vi "ScreeningPlatform_v4.vi"() -> ()   [LabVIEW 2018]
uses:
  <instrlib>/Chemyx/_driver/Basic driver/Communication/controls/comm_rate_enum.ctl
  <vilib>/Utility/file.llb/Read Delimited Spreadsheet (DBL).vi
  <vilib>/Utility/file.llb/Read Delimited Spreadsheet (string).vi
  <vilib>/regexp/Match Regular Expression.xnode
  <instrlib>/Chemyx/_driver/Chemyx_Syringe_Pump_driver.lvlib
panel:
  out "Start Scan":dbl format="%#_1f"
  out "Stop Scan":dbl format="%#_1f"
  in  "stop":bool
  in  "GPC Injections":bool=TRUE
  out "Comments file":path=path "Z:/Sci-Chem/PRD/NMR 112/Automated Platform/2020/08/17/332PM_JOreneosdjf/Software Details/JOreneosdjf_Comments.txt"
  in  "Insert Comment":bool
  in  "Cooment":string
  out "NMR use":bool
  out "GPC use":bool
  out "GPC Dead Volume":bool
  out "GPC timesweep":bool
  out "NMR timesweep":bool
  out "NMR Dead Volume":bool
  out "Stabilisation":bool
  out "OverviewTextFile":path=path "Z:/Sci-Chem/PRD/NMR 112/Automated Platform/2020/08/17/332PM_JOreneosdjf/Software Details/JOreneosdjf_OverviewText.txt"
  out "To... (min)":dbl
  out "From.. (min)":dbl
  out "Dead Volume 3":dbl
  out "Dilution Flowrate":dbl
  out "NMR interval":dbl
  out "Dead Volume 1":dbl
  out "Stabilisation Factor":dbl
  out "Reactor Volume":dbl
  out "Dead Volume 2":dbl
  out "GPC interval":dbl
  out "TimesweepStringArray":string[][](array[string])=[["1.0", "5.0", "1.0", "1.0", "0.2", "1.3", "0.43", "0.26", "3", "0.157", "1.5", "2.15", "1.3", "0.10466666666666667", "15", "GPCandNMR"]]
  out "Experiment started":bool
  out "Experiment folder created":bool
  out "Experiment found":bool
  in  "Tab Control":enum32{"Overview", "Details", "Folders"}(tab)=enum."Folders"
  in  "Listbox":i32(listbox)
  in  "Finished_timesweeps":i32(listbox)=-1
  out "Timesweep queue":string[](array[string])=["Timesweep 1: From 1.0 minutes (1.000 mL/min) to 5.0 minutes (0.200 mL/min) with GPC intervals of 3.0 minutes."]
  out "Content Textfile":string
  out "Experiment Folder (path)":path=path "Z:/Sci-Chem/PRD/NMR 112/Automated Platform/2020/09/30/936AM_2"
  out "Mode":string
  out "TimesweepArray":dbl[][](array[numeric])
  out "Last Comment":string
  in  "Python Communication Folder":path=path "S:/Sci-Chem/PRD/NMR 112/Automated Platform/Final_LabView_allVIs/PythonCommunication"
  in  "Where to save?":path=path "S:/Sci-Chem/PRD/NMR 112/Automated Platform"
  out "Status injections":string="Waiting for injection 0"
  out "NAME":string="No new experiment found..."
  out "output array":dbl[](array[numeric])=[5.0, 17.0]
  out "Reaction":dbl[][](array[numeric])
  out "Next injection":u8(slide) scale=0.0..100.0
  out "GPC Samples":dbl format="%#_1f"
  in  "GPC connection port 2":refnum<visa-resource-name>
  in  "Pump":refnum<visa-resource-name>="COM11"
  out "Waiting NMR":dbl format="%#_2g"
  out "Waiting GPC":dbl format="%#_2f"
  out "scan":i32
  out "GPC Status":string
  out "NMR Status":string
  out "Current timesweep":i32
  out "Stabilisation time (min)":dbl=nan format="%#_2g"
  out "Stabilisation time (sec)":dbl=nan
  out "GPC Timesweep":u8(slide) scale=0.0..100.0
  out "NMR Timesweep bar":u8(slide) scale=0.0..100.0
  out "StabilisationBar":u8(slide) scale=0.0..100.0
  out "Status":string="Start program..."
  # "Reactor Volume"
  # "mL"
  # "Dead Volume 2"
  # "mL"
  # "Dead Volume 1"
  # "mL"
  # "Dead Volume 3"
  # "mL"
  # "Stabilisation Factor"
  # "x"
  # "Dilution Flowrate"
  # "mL/min"
  # "NMR interval"
  # "sec"
  # "GPC interval"
  # "min"
  # "Stabilisation"
  # "min"
  # "Use"
  # "Dead Volume"
  # "Timesweep"
  # "Done"
  # "Status"
  # "Number"
  # "min"
  # "NMR"
  # "min"
  # "GPC"
  # "Next injection"
  # "Comment"
  # "scan"
  # "to"
  # "Experiment found"
  # "Experiment folder created"
  # "Experiment started"
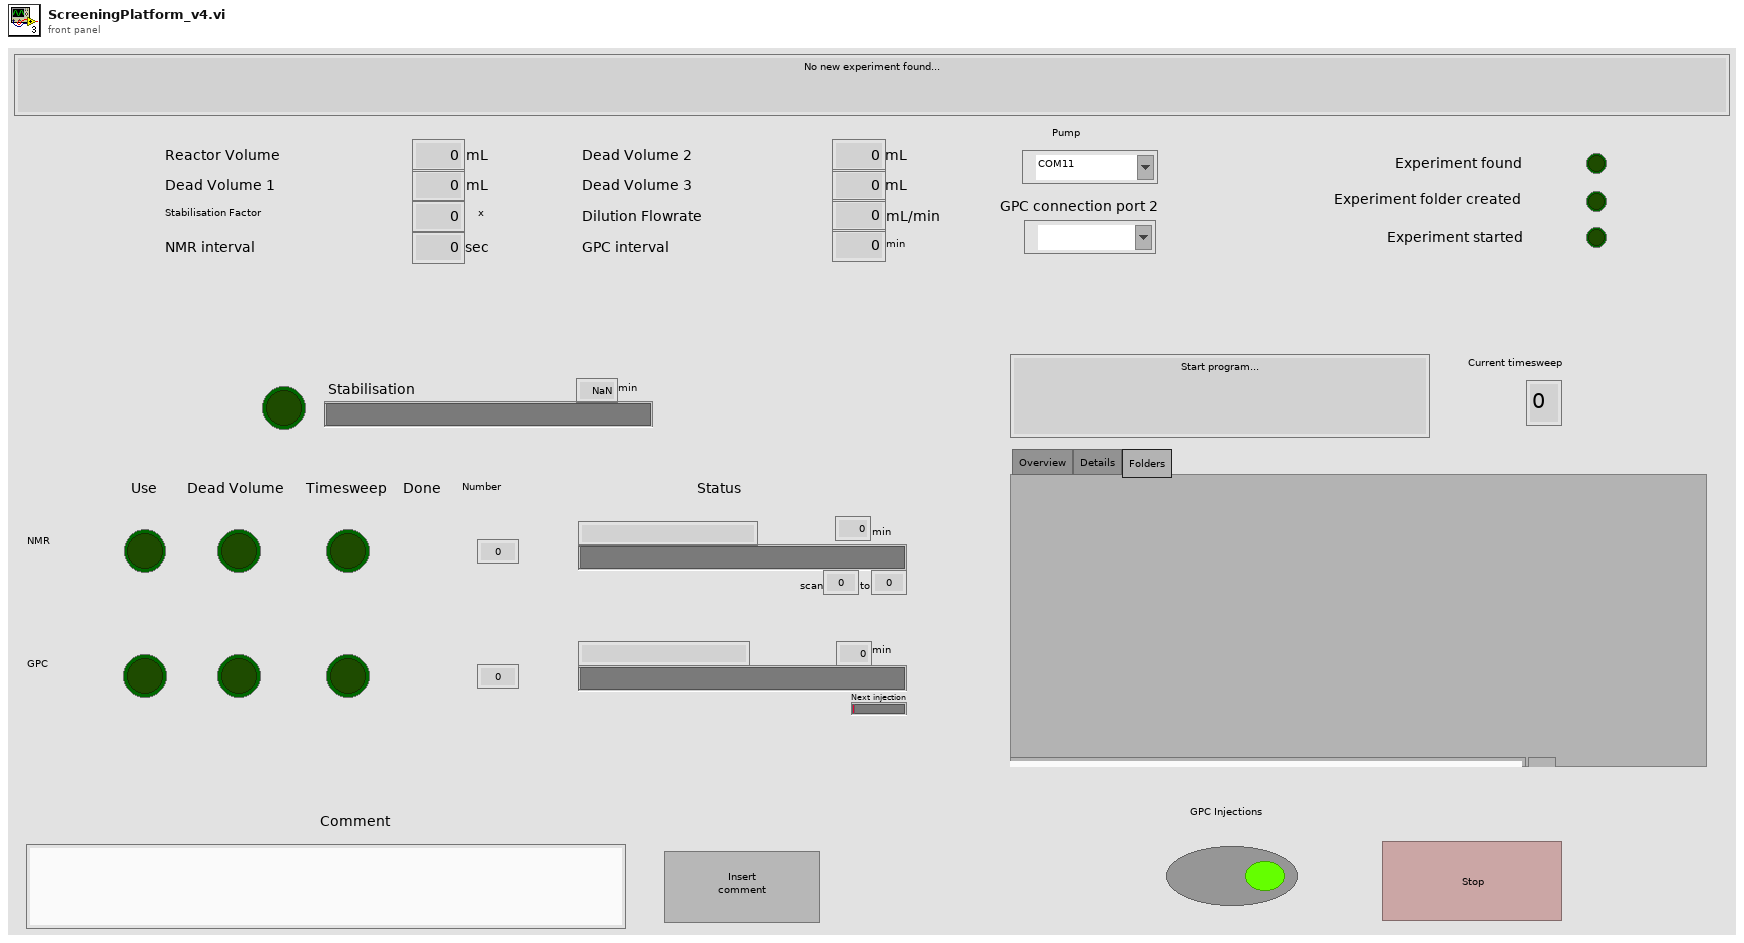
[diagram p1: front panel]
types:
  T1 = typedef "Chemyx_Syringe_Pump_driver.lvlib/comm_rate_enum.ctl" = enum16{"9600", "38400"}
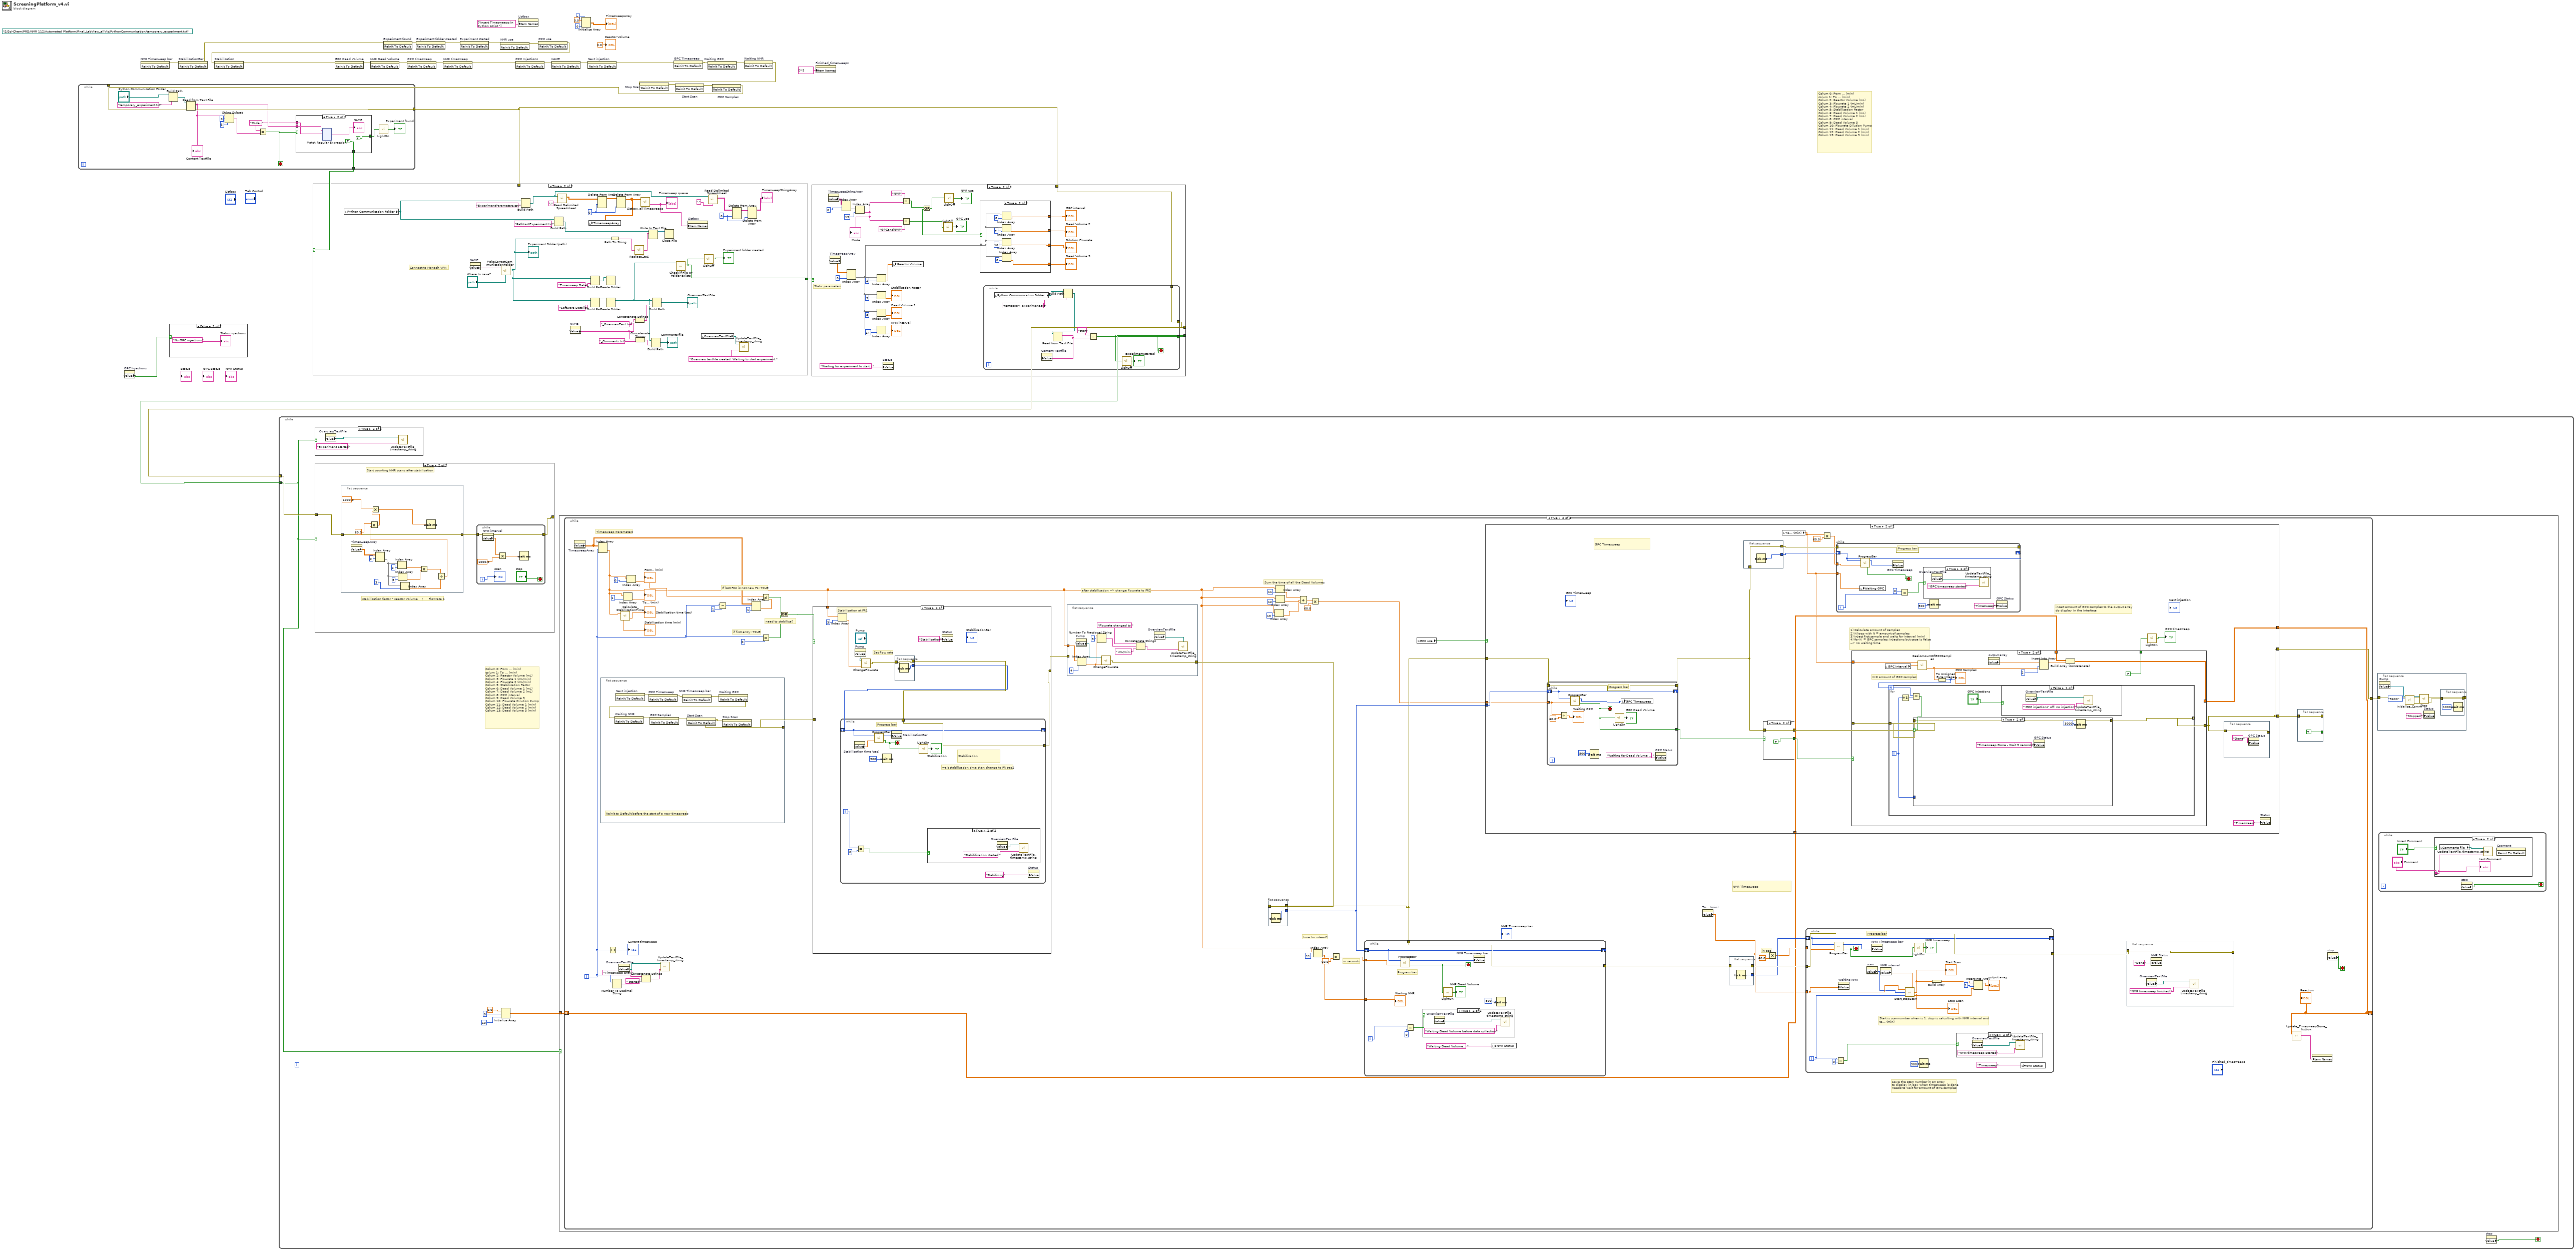
[diagram p0: block diagram]
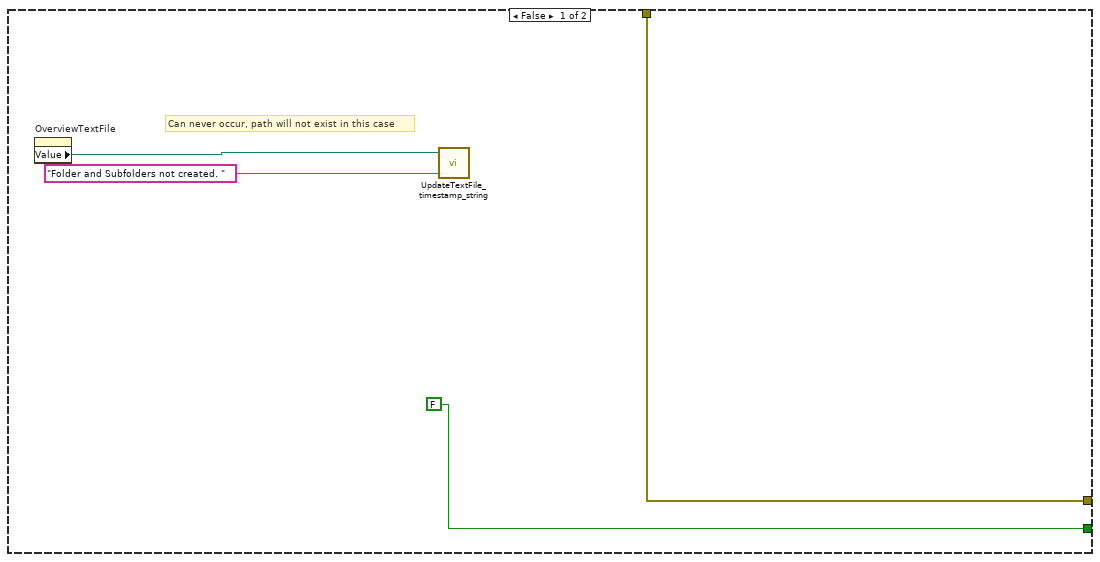
[diagram p3: hidden frame]
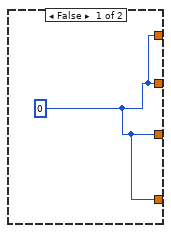
[diagram p4: hidden frame]
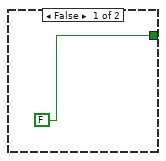
[diagram p5: hidden frame]
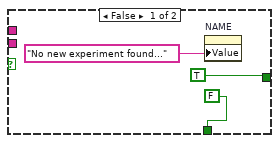
[diagram p6: hidden frame]
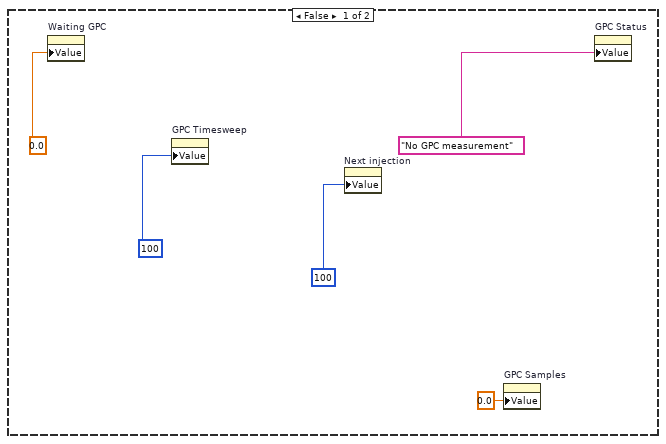
[diagram p11: hidden frame]
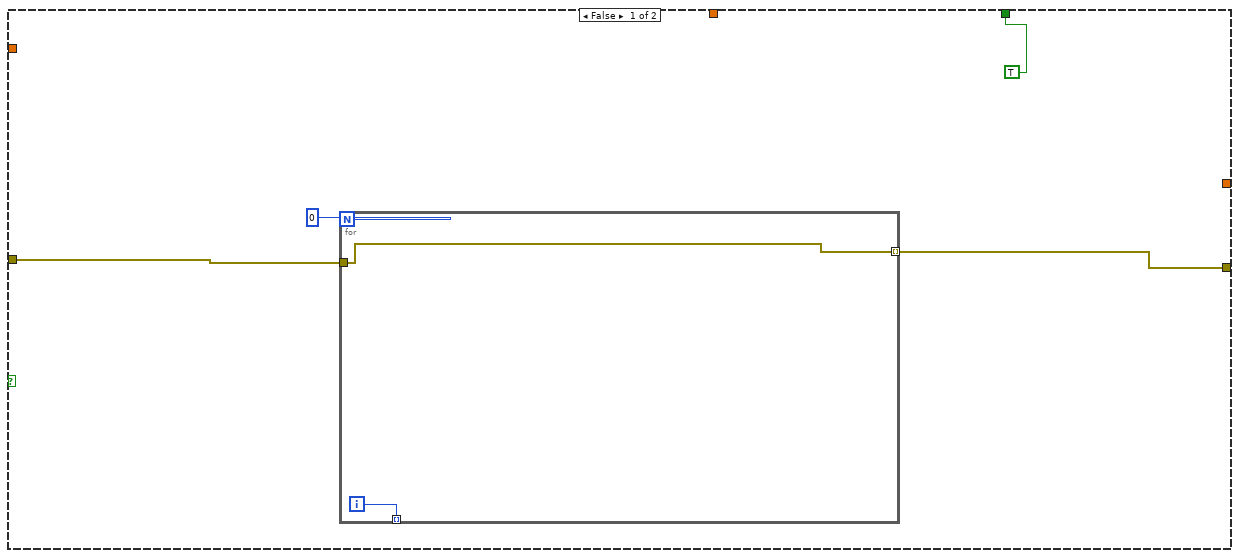
[diagram p12: hidden frame]
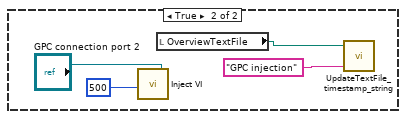
[diagram p13: hidden frame]
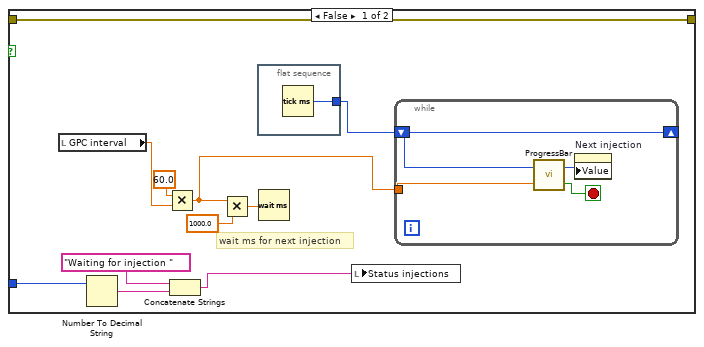
[diagram p14: hidden frame]
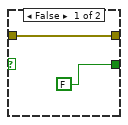
[diagram p16: hidden frame]
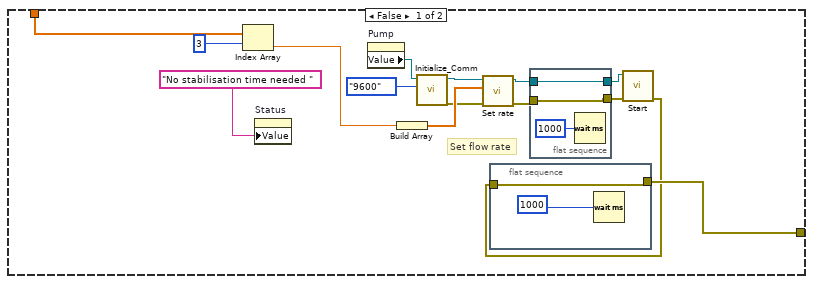
[diagram p18: hidden frame]
diagram:
  (unwired) path "S:/Sci-Chem/PRD/NMR 112/Automated Platform/Final_LabView_allVIs/PythonCommunication/temporary_experiment.txt" ("file path (dialog if empty)")
  # "Colum 0: From ... (min)\ncolum 1: To ... (min)\nColum 2: Reactor Volume (mL)\nColum 3: Flowrate 1 (mL/min)\nColum 4: Flowrate 2 (mL/min)\nColum 5: Stabilisation Factor\nColum 6: Dead Volume 1 (mL)\nColum 7: Dead Volume 2 (mL)\nColum 8: GPC interval\nColum 9: Dead Volume 3\nColum 10: Flowrate Dilution Pump\nColum 11: Dead Volume 1 (min)\nColum 12: Dead Volume 2 (min)\nColum 13: Dead Volume 3 (min)"
  n1 = property on="GPC Injections" class="Bool (strict)"() -> ("Value"=w28:bool)  [unwired: 2 in, 2 out]
  n2 = invoke on="NMR Timesweep bar" class="Slide (strict)" method="Reinit To Default"() -> (error out=w30:errorcluster)  [unwired: 3 in, 2 out]
  n3 = case shown="False" w28 {
    frame False {
      "Status injections" <- "No GPC injections"
    }
    frame True {
    }
  }
  n4 = invoke on="StabilisationBar" class="Slide (strict)" method="Reinit To Default"(error in=w30) -> (error out=w25:errorcluster)  [unwired: 2 in, 2 out]
  n5 = invoke on="Experiment found" class="Bool (strict)" method="Reinit To Default"(error in=w25) -> (error out=w27:errorcluster)  [unwired: 2 in, 2 out]
  n6 = invoke on="Experiment folder created" class="Bool (strict)" method="Reinit To Default"(error in=w27) -> (error out=w26:errorcluster)  [unwired: 2 in, 2 out]
  n7 = invoke on="Experiment started" class="Bool (strict)" method="Reinit To Default"(error in=w26) -> (error out=w3:errorcluster)  [unwired: 2 in, 2 out]
  n8 = invoke on="NMR use" class="Bool (strict)" method="Reinit To Default"(error in=w3) -> (error out=w2:errorcluster)  [unwired: 2 in, 2 out]
  n9 = property on="Listbox" class="LstBox (strict)"("Item Names"=string[] ["Insert Timesweeps in Python script "]) -> ()  [unwired: 2 in, 2 out]
  n10 = invoke on="GPC use" class="Bool (strict)" method="Reinit To Default"(error in=w2) -> (error out=w1:errorcluster)  [unwired: 2 in, 2 out]
  n11 = invoke on="Stabilisation" class="Bool (strict)" method="Reinit To Default"(error in=w1) -> (error out=w24:errorcluster)  [unwired: 2 in, 2 out]
  n12 = invoke on="GPC Dead Volume" class="Bool (strict)" method="Reinit To Default"(error in=w24) -> (error out=w23:errorcluster)  [unwired: 2 in, 2 out]
  n13 = invoke on="NMR Dead Volume" class="Bool (strict)" method="Reinit To Default"(error in=w23) -> (error out=w22:errorcluster)  [unwired: 2 in, 2 out]
  n14 = invoke on="GPC timesweep" class="Bool (strict)" method="Reinit To Default"(error in=w22) -> (error out=w21:errorcluster)  [unwired: 2 in, 2 out]
  n15 = invoke on="NMR timesweep" class="Bool (strict)" method="Reinit To Default"(error in=w21) -> (error out=w18:errorcluster)  [unwired: 2 in, 2 out]
  n16 = invoke on="GPC Injections" class="Bool (strict)" method="Reinit To Default"(error in=w18) -> (error out=w20:errorcluster)  [unwired: 2 in, 2 out]
  n17 = invoke on="NAME" class="Str" method="Reinit To Default"(error in=w20) -> (error out=w19:errorcluster)  [unwired: 2 in, 2 out]
  n18 = Initialize Array(0.0 ("element"), 0 ("dimension size"), 0 ("dimension size")) -> (→"TimesweepArray":dbl[][])
  n19 = invoke on="Next injection" class="Slide (strict)" method="Reinit To Default"(error in=w19) -> (error out=w13:errorcluster)  [unwired: 2 in, 2 out]
  n20 = invoke on="GPC Timesweep" class="Slide (strict)" method="Reinit To Default"(error in=w13) -> (error out=w15:errorcluster)  [unwired: 2 in, 2 out]
  n21 = invoke on="Waiting GPC" class="DigNum (strict)" method="Reinit To Default"(error in=w15) -> (error out=w16:errorcluster)  [unwired: 2 in, 2 out]
  n22 = invoke on="Waiting NMR" class="DigNum (strict)" method="Reinit To Default"(error in=w16) -> (error out=w12:errorcluster)  [unwired: 2 in, 2 out]
  n23 = invoke on="Stop Scan" class="DigNum (strict)" method="Reinit To Default"(error in=w12) -> (error out=w17:errorcluster)  [unwired: 2 in, 2 out]
  n24 = invoke on="Start Scan" class="DigNum (strict)" method="Reinit To Default"(error in=w17) -> (error out=w14:errorcluster)  [unwired: 2 in, 2 out]
  n25 = invoke on="GPC Samples" class="DigNum (strict)" method="Reinit To Default"(error in=w14) -> (error out=w11:errorcluster)  [unwired: 2 in, 2 out]
  n26 = while {
    tunnel: [w49] -> w34
    tunnel: w11 -> [w42]
    tunnel: [w41] -> w29
    stop <- w45 stop-if-true
    w43 = "Code,," ("y")
    n27 = Build Path(base path="Python Communication Folder", name or relative path="temporary_experiment.txt") -> (appended path=w36:path)
    n28 = Read from Text File(file (use dialog)=w36, error in=w42) -> (text=w44:string, error out=w49:errorcluster)  [unwired: 2 in, 2 out]
    "Content Textfile" <- w44
    n29 = String Subset(string=w44, offset (0)=0, length (rest)=6 ("length (rest)")) -> (substring=w46:string)
    n30 = Equal?(x=w43, y=w46) -> (x = y?=w45:bool)
    n31 = case shown="True" w45 {
      tunnel: w44 -> [_ w57]
      tunnel: w43 -> [_ w56]
      tunnel: [FALSE TRUE] -> w41
      tunnel: [TRUE FALSE] -> w40
      frame False {
        n32 = property on="NAME" class="Str"("Value"="No new experiment found...") -> ()  [unwired: 2 in, 2 out]
      }
      frame True {
        n33 = xnode "Match Regular Expression"("input string"=w57, "regular expression"=w56) -> ("after match"=→"NAME":string)  [unwired: 4 in, 4 out]
      }
    }
    n34 = call "LightOn.vi"("Turns off when..."=w40) -> ("Light Indicator"=→"Experiment found":bool)
  }
  n35 = case shown="True" w29 {
    tunnel: w34 -> [_ _]
    tunnel: [FALSE w198] -> w31
    frame False {
    }
    frame True {
      w191 = 0 ("index (row)")
      w208 = 0 ("length")
      # "Connect to Monash VPN"
      n36 = local read "Python Communication Folder"() -> (w177:path)
      n37 = property on="NAME" class="Str"() -> ("Value"=w203:string)  [unwired: 2 in, 2 out]
      n38 = call "MakeCorrectCommunicationFolder.vi"("Main_dataFolder"="Where to save?", "SampleName"=w203) -> ("Communication Folder"=w182:path)  [unwired: 1 out]
      "Experiment Folder (path)" <- w182
      n39 = Build Path(base path=w177, name or relative path="ExperimentParameters.csv") -> (appended path=w179:path)
      n40 = Build Path(base path=w177, name or relative path="PathLastExperiment.txt") -> (appended path=w180:path)
      n41 = call-poly <vilib>:"Read Delimited Spreadsheet.vi"("file path (dialog if empty)"=w179, "delimiter (\\t)"="," ("delimiter (\\t)")) -> ("all rows"=w207:dbl[][])  [unwired: 8 in, 5 out]
      n42 = property on="NAME" class="Str"() -> ("Value"=w188:string)  [unwired: 2 in, 2 out]
      n43 = Build Path(base path=w182, name or relative path="Timesweep Data") -> (appended path=w199:path)
      n44 = Build Path(base path=w182, name or relative path="Software Details") -> (appended path=w200:path)
      n45 = Delete From Array(array=w207, index (row)=w208) -> (array with subset deleted=w209:dbl[][])  [unwired: 2 in, 1 out]
      n46 = Create Folder(path (use dialog)=w199) -> ()  [unwired: 2 in, 3 out]
      n47 = Create Folder(path (use dialog)=w200) -> (created path=w189:path)  [unwired: 2 in, 2 out]
      n48 = Path To String(path=w182) -> (string=w175:string)
      n49 = Delete From Array(array=w209, index (col)=w208) -> (array with subset deleted=w183:dbl[][])  [unwired: 2 in, 1 out]
      n50 = local write "TimesweepArray"(w183) -> ()
      n51 = call "ReplaceZtoS.vi"("String"=w175) -> ("result string"=w174:string)
      n52 = Concatenate Strings(w188, "_OverviewText.txt" ("string")) -> (w201:string)
      n53 = Concatenate Strings(w188, "_Comments.txt" ("string")) -> (w186:string)
      n54 = call "Listbox_allTimesweeps.vi"("new array"=w183) -> ("output array"=w184:string[])  [unwired: 1 out]
      "Timesweep queue" <- w184
      n55 = Write to Text File(file (use dialog)=w180, text=w174) -> (refnum out=w205:refnum<file>)  [unwired: 2 in, 2 out]
      n56 = Build Path(base path=w189, name or relative path=w186) -> (appended path=→"Comments file":path)
      n57 = Build Path(base path=w189, name or relative path=w201) -> (appended path=→"OverviewTextFile":path)
      n58 = Close File(refnum=w205) -> ()  [unwired: 1 in, 2 out]
      n59 = call <vilib>:"Check if File or Folder Exists.vi"("path"=w189) -> ("file or folder exists?"=w198:bool)  [unwired: 8 in, 2 out]
      n60 = property on="Listbox" class="LstBox (strict)"("Item Names"=w184) -> ()  [unwired: 2 in, 2 out]
      n61 = local read "OverviewTextFile"() -> (w173:path)
      n62 = call "LighOff.vi"("Turns on when..."=w198) -> ("Light Indicator"=→"Experiment folder created":bool)
      n63 = call-poly <vilib>:"Read Delimited Spreadsheet.vi"("file path (dialog if empty)"=w179, "delimiter (\\t)"="," ("delimiter (\\t)")) -> ("all rows"=w194:string[][])  [unwired: 8 in, 5 out]
      n64 = Delete From Array(array=w194, index (row)=w191) -> (array with subset deleted=w193:string[][])  [unwired: 2 in, 1 out]
      n65 = call "UpdateTextFile_timestamp_string.vi"("string"="Overview textfile created. Waiting to start experiment.", "file path"=w173) -> ()  [unwired: 1 in]
      n66 = Delete From Array(array=w193, index (col)=w191) -> (array with subset deleted=→"TimesweepStringArray":string[][])  [unwired: 2 in, 1 out]
    }
  }
  n67 = case shown="True" w31 {
    tunnel: [w214 w245] -> w33
    tunnel: [FALSE w244] -> w32
    tunnel: w34 -> [w214 w243]
    frame False {
      # "Can never occur, path will not exist in this case"
      n68 = property on="OverviewTextFile" class="Path"() -> ("Value"=w212:path)  [unwired: 2 in, 2 out]
      n69 = call "UpdateTextFile_timestamp_string.vi"("string"="Folder and Subfolders not created. ", "file path"=w212) -> ()  [unwired: 1 in]
    }
    frame True {
      # "Static parameters"
      n70 = property on="TimesweepStringArray" class="Arr (strict)"() -> ("Value"=w234:string[][])  [unwired: 2 in, 2 out]
      n71 = property on="TimesweepArray" class="Arr (strict)"() -> ("Value"=w241:dbl[][])  [unwired: 2 in, 2 out]
      n72 = Index Array(array=w234, index (row)=0 ("disabled index (col)")) -> (element=w233:string[])  [unwired: 1 in]
      n73 = Index Array(array=w241, index (row)=0) -> (element=w221:dbl[])  [unwired: 1 in]
      n74 = Index Array(array=w233, index=15) -> (element=w216:string)
      "Mode" <- w216
      n75 = Index Array(array=w221, index=2) -> (element=w215:dbl)
      n76 = Index Array(array=w221, index=5) -> (element=→"Stabilisation Factor":dbl)
      n77 = Index Array(array=w221, index=6) -> (element=→"Dead Volume 1":dbl)
      n78 = Index Array(array=w221, index=14) -> (element=→"NMR interval":dbl)
      n79 = property on="Status" class="Str"("Value"="Waiting for experiment to start..." ("Status")) -> ()  [unwired: 2 in, 2 out]
      n80 = local write "Reactor Volume"(w215) -> ()
      n81 = Equal?(x="NMR", y=w216) -> (x = y?=w225:bool)
      n82 = Equal?(x=w216, y="GPCandNMR") -> (x = y?=w222:bool)
      n83 = Or(x=w225, y=w222) -> (x .or. y?=w228:bool)
      n84 = call "LighOff.vi"("Turns on when..."=w222) -> ("Light Indicator"=→"GPC use":bool)
      n85 = call "LighOff.vi"("Turns on when..."=w228) -> ("Light Indicator"=→"NMR use":bool)
      n86 = case shown="True" w222 {
        tunnel: w221 -> [_ w251]
        tunnel: [w246 w254] -> w224
        tunnel: [w246 w253] -> w223
        tunnel: [w246 w250] -> w218
        tunnel: [w246 w249] -> w217
        frame False {
          w246 = 0
        }
        frame True {
          n87 = Index Array(array=w251, index=8) -> (element=w254:dbl)
          n88 = Index Array(array=w251, index=7) -> (element=w253:dbl)
          n89 = Index Array(array=w251, index=10) -> (element=w250:dbl)
          n90 = Index Array(array=w251, index=8) -> (element=w249:dbl)
        }
      }
      "GPC interval" <- w224
      "Dead Volume 2" <- w223
      "Dilution Flowrate" <- w218
      "Dead Volume 3" <- w217
      n91 = while {
        tunnel: [w262] -> w245
        tunnel: w243 -> [w262]
        tunnel: [w260] -> w244
        stop <- w260 stop-if-true
        n92 = local read "Python Communication Folder"() -> (w258:path)
        n93 = Build Path(base path=w258, name or relative path="temporary_experiment.txt") -> (appended path=w256:path)
        n94 = Read from Text File(file (use dialog)=w256) -> (text=w261:string)  [unwired: 3 in, 3 out]
        n95 = property on="Content Textfile" class="Str"("Value"=w261) -> ()  [unwired: 2 in, 2 out]
        n96 = Equal?(x="start" ("y"), y=w261) -> (x = y?=w260:bool)
        n97 = call "LighOff.vi"("Turns on when..."=w260) -> ("Light Indicator"=→"Experiment started":bool)
      }
    }
  }
  n98 = while {
    tunnel: w33 -> [w266]
    tunnel: w32 -> [w265]
    stop <- w264 stop-if-true
    # "Colum 0: From ... (min)\ncolum 1: To ... (min)\nColum 2: Reactor Volume (mL)\nColum 3: Flowrate 1 (mL/min)\nColum 4: Flowrate 2 (mL/min)\nColum 5: Stabilisation Factor\nColum 6: Dead Volume 1 (mL)\nColum 7: Dead Volume 2 (mL)\nColum 8: GPC interval\nColum 9: Dead Volume 3\nColum 10: Flowrate Dilution Pump\nColum 11: Dead Volume 1 (min)\nColum 12: Dead Volume 2 (min)\nColum 13: Dead Volume 3 (min)"
    n99 = case shown="True" w265 {
      frame False {
      }
      frame True {
        n100 = property on="OverviewTextFile" class="Path"() -> ("Value"=w271:path)  [unwired: 2 in, 2 out]
        n101 = call "UpdateTextFile_timestamp_string.vi"("string"="Experiment Started", "file path"=w271) -> ()  [unwired: 1 in]
      }
    }
    n102 = case shown="True" w265 {
      tunnel: w266 -> [w273 w276]
      tunnel: [w273 w274] -> _
      frame False {
      }
      frame True {
        # "Start counting NMR scans after stabilisation"
        # "stabilisation factor * reactor Volume    /      Flowrate 1"
        n103 = flat-sequence {
          tunnel: w276 -> [w281]
          tunnel: [w281] -> w275
          frame #0 {
            n104 = property on="TimesweepArray" class="Arr (strict)"() -> ("Value"=w277:dbl[][])  [unwired: 2 in, 2 out]
            n105 = Index Array(array=w277, index (row)=0) -> (element=w282:dbl[])  [unwired: 1 in]
            n106 = Index Array(array=w282, index=2) -> (element=w290:dbl)
            n107 = Index Array(array=w282, index=5) -> (element=w291:dbl)
            n108 = Index Array(array=w282, index=3) -> (element=w283:dbl)
            n109 = Multiply(x=w290, y=w291) -> (x*y=w292:dbl)
            n110 = Divide(x=w292, y=w283) -> (x/y=w280:dbl)
            n111 = Multiply(x=60.0 ("y"), y=w280) -> (x*y=w278:dbl)
            n112 = Multiply(x=1000.0, y=w278) -> (x*y=w284:dbl)
            n113 = Wait (ms)(milliseconds to wait=w284) -> ()  [unwired: 1 out]
          }
        }
        n114 = while {
          tunnel: w275 -> [w297]
          tunnel: [w297] -> w274
          i -> [w298]
          stop <- "stop" stop-if-true
          n115 = property on="NMR interval" class="DigNum (strict)"() -> ("Value"=w293:dbl)  [unwired: 2 in, 2 out]
          n116 = Multiply(x=w293, y=1000.0) -> (x*y=w296:dbl)
          n117 = Wait (ms)(milliseconds to wait=w296) -> ()  [unwired: 1 out]
          "scan" <- w298
        }
      }
    }
    n118 = Initialize Array(0.0 ("element"), 0 ("dimension size"), 10 ("dimension size")) -> (w267:dbl[][])
    n119 = case shown="True" w265 {
      tunnel: w267 -> [_ w299]
      frame False {
      }
      frame True {
        n120 = while {
          tunnel: [w317] -> w300
          shift-right: [w346] -> _
          shift-left: w299 -> [w347]
          i -> [w321]
          stop <- w330 stop-if-true
          # "Save the scan number in an array\nto display in box when timesweep is done\nneeds to wait for amount of GPC samples"
          # "time for vdead1"
          # "Timesweep Parameters"
          # "in sec"
          # "in seconds"
          # "Sum the time of all the Dead Volumes"
          # "after stabilisation --> change flowrate to FR2"
          # "If last FR2 is not new F1: TRUE"
          # "if first entry: TRUE"
          # "need to stabilize?"
          # "NMR Timesweep"
          n121 = property on="TimesweepArray" class="Arr (strict)"() -> ("Value"=w328:dbl[][])  [unwired: 2 in, 2 out]
          n122 = Index Array(array=w328, index (row)=w321) -> (element=w325:dbl[])  [unwired: 1 in]
          n123 = flat-sequence {
            tunnel: [w489] -> w315
            frame #0 {
              # "Reinit to Default before the start of a new timesweep"
              n124 = invoke on="Next injection" class="Slide (strict)" method="Reinit To Default"() -> (error out=w490:errorcluster)  [unwired: 3 in, 2 out]
              n125 = invoke on="GPC Timesweep" class="Slide (strict)" method="Reinit To Default"(error in=w490) -> (error out=w491:errorcluster)  [unwired: 2 in, 2 out]
              n126 = invoke on="NMR Timesweep bar" class="Slide (strict)" method="Reinit To Default"(error in=w491) -> (error out=w492:errorcluster)  [unwired: 2 in, 2 out]
              n127 = invoke on="Waiting GPC" class="DigNum (strict)" method="Reinit To Default"(error in=w492) -> (error out=w493:errorcluster)  [unwired: 2 in, 2 out]
              n128 = invoke on="Waiting NMR" class="DigNum (strict)" method="Reinit To Default"(error in=w493) -> (error out=w494:errorcluster)  [unwired: 2 in, 2 out]
              n129 = invoke on="GPC Samples" class="DigNum (strict)" method="Reinit To Default"(error in=w494) -> (error out=w487:errorcluster)  [unwired: 2 in, 2 out]
              n130 = invoke on="Start Scan" class="DigNum (strict)" method="Reinit To Default"(error in=w487) -> (error out=w488:errorcluster)  [unwired: 2 in, 2 out]
              n131 = invoke on="Stop Scan" class="DigNum (strict)" method="Reinit To Default"(error in=w488) -> (error out=w489:errorcluster)  [unwired: 2 in, 2 out]
            }
          }
          n132 = Increment(x=w321) -> (x+1=→"Current timesweep":i32)
          n133 = Number To Decimal String(number=w321) -> (decimal integer string=w322:string)  [unwired: 1 in]
          n134 = property on="OverviewTextFile" class="Path"() -> ("Value"=w323:path)  [unwired: 2 in, 2 out]
          n135 = call "Calculate_StabilisationTime.vi"("New Array"=w325) -> ("Stabilisation time (sec)"=→"Stabilisation time (sec)":dbl, "Stabilisation time (min)"=→"Stabilisation time (min)":dbl)  [unwired: 1 in]
          n136 = Index Array(array=w325, index=1) -> (element=→"To... (min)":dbl)
          n137 = Index Array(array=w325, index=0) -> (element=w326:dbl)
          "From.. (min)" <- w326
          n138 = Concatenate Strings("Timesweep entry" ("string"), w322, " started" ("string")) -> (w318:string)
          n139 = call "UpdateTextFile_timestamp_string.vi"("string"=w318, "file path"=w323) -> ()  [unwired: 1 in]
          n140 = Subtract(x=w321, y=1) -> (x-y=w358:i32)
          n141 = Index Array(array=w328, index (row)=w358, index (col)=1) -> (element=w357:dbl)
          n142 = Not Equal?(x=w326, y=w357) -> (x != y?=w362:bool)
          n143 = Equal?(x=w321, y=0) -> (x = y?=w363:bool)
          n144 = Or(x=w362, y=w363) -> (x .or. y?=w361:bool)
          n145 = case shown="True" w361 {
            tunnel: [w525 w548] -> w368
            tunnel: w325 -> [w526 w547]
            tunnel: w315 -> [_ _]
            frame False {
              # "Set flow rate"
              n146 = Index Array(array=w526, index=3) -> (element=w532:dbl)
              n147 = property on="Status" class="Str"("Value"="No stabilisation time needed " ("Status")) -> ()  [unwired: 2 in, 2 out]
              n148 = property on="Pump" class="VISAName"() -> ("Value"=w522:refnum<visa-resource-name>)  [unwired: 2 in, 2 out]
              n149 = Build Array(w532) -> (w531:dbl[])
              n150 = call <instrlib>:"Initialize_Comm.vi"("Baud rate"=comm_rate_enum."9600", "Serial Port in"=w522) -> ("error out"=w529:errorcluster, "Serial Port out"=w530:refnum<visa-resource-name>)  [unwired: 8 in]
              n151 = call <instrlib>:"Set rate.vi"("error in (no error)"=w529, "Rate (array)"=w531, "Serial Port in"=w530) -> ("error out"=w536:errorcluster, "Serial Port out"=w533:refnum<visa-resource-name>)  [unwired: 7 in]
              n152 = flat-sequence {
                tunnel: [w538] -> w525
                tunnel: w523 -> [w538]
                frame #0 {
                  n153 = Wait (ms)(milliseconds to wait=u32 1000 ("millisecond timer value")) -> ()  [unwired: 1 out]
                }
              }
              n154 = flat-sequence {
                tunnel: w533 -> [w541]
                tunnel: [w541] -> w534
                tunnel: w536 -> [w540]
                tunnel: [w540] -> w535
                frame #0 {
                  n155 = Wait (ms)(milliseconds to wait=u32 1000) -> ()  [unwired: 1 out]
                }
              }
              n156 = call <instrlib>:"Start.vi"("error in (no error)"=w535, "Serial Port in"=w534) -> ("error out"=w523:errorcluster)  [unwired: 8 in, 1 out]
            }
            frame True {
              # "Stabilisation at FR1"
              # "Set flow rate"
              n157 = Index Array(array=w547, index=3) -> (element=w544:dbl)
              n158 = while {
                shift-right: [w560] -> _
                shift-left: w546 -> [w560]
                tunnel: w549 -> [w562]
                tunnel: [w562] -> w548
                i -> [w553]
                stop <- w555 stop-if-true
                # "wait stabilisation time then change to FR tres2"
                # "Stabilisation"
                # "Progress bar"
                n159 = property on="Stabilisation time (sec)" class="DigNum (strict)"() -> ("Value"=w559:dbl)  [unwired: 2 in, 2 out]
                n160 = Equal?(x=w553, y=0) -> (x = y?=w556:bool)
                n161 = call "ProgressBar.vi"("Time_end"=w559, "TimeBegin"=w560) -> ("TrueFalse"=w555:bool, "Stabilisation Bar"=w558:u8)
                n162 = Wait (ms)(milliseconds to wait=u32 500) -> ()  [unwired: 1 out]
                n163 = property on="StabilisationBar" class="Slide (strict)"("Value"=w558) -> ()  [unwired: 2 in, 2 out]
                n164 = call "LightOn.vi"("Turns off when..."=w555) -> ("Light Indicator"=→"Stabilisation":bool)
                n165 = case shown="True" w556 {
                  frame False {
                  }
                  frame True {
                    n166 = property on="OverviewTextFile" class="Path"() -> ("Value"=w564:path)  [unwired: 2 in, 2 out]
                    n167 = call "UpdateTextFile_timestamp_string.vi"("string"="Stabililisation started ", "file path"=w564) -> ()  [unwired: 1 in]
                  }
                }
                n168 = property on="Status" class="Str"("Value"="Stabilising" ("Status")) -> ()  [unwired: 2 in, 2 out]
              }
              n169 = property on="Pump" class="VISAName"() -> ("Value"=w545:refnum<visa-resource-name>)  [unwired: 2 in, 2 out]
              n170 = call "ChangeFlowrate.vi"("Flowrate"=w544, "Serial Port in"=w545) -> ("error out"=w543:errorcluster)
              n171 = flat-sequence {
                tunnel: [w552] -> w546
                tunnel: [w551] -> w549
                tunnel: w543 -> [w551]
                frame #0 {
                  n172 = Tick Count (ms)() -> (millisecond timer value=w552:u32)
                }
              }
              n173 = property on="Status" class="Str"("Value"="Stabilisation" ("Status")) -> ()  [unwired: 2 in, 2 out]
            }
          }
          n174 = flat-sequence {
            tunnel: [w482] -> w369
            tunnel: w368 -> [_]
            tunnel: w325 -> [w486]
            frame #0 {
              n175 = property on="Pump" class="VISAName"() -> ("Value"=w483:refnum<visa-resource-name>)  [unwired: 2 in, 2 out]
              n176 = Index Array(array=w486, index=4) -> (element=w478:dbl)
              n177 = Number To Fractional String(number=w478, precision (6)=i16 3 ("width (-)")) -> (F-format string=w477:string)  [unwired: 2 in]
              n178 = call "ChangeFlowrate.vi"("Flowrate"=w478, "Serial Port in"=w483) -> ("error out"=w482:errorcluster)
              n179 = Concatenate Strings("Flowrate changed to " ("string"), w477, " mL/min." ("string")) -> (w479:string)
              n180 = property on="OverviewTextFile" class="Path"() -> ("Value"=w484:path)  [unwired: 2 in, 2 out]
              n181 = call "UpdateTextFile_timestamp_string.vi"("string"=w479, "file path"=w484) -> ()  [unwired: 1 in]
            }
          }
          n182 = flat-sequence {
            tunnel: [w581] -> w367
            tunnel: [w580] -> w366
            tunnel: w369 -> [w580]
            frame #0 {
              n183 = Tick Count (ms)() -> (millisecond timer value=w581:u32)
            }
          }
          n184 = Index Array(array=w325, index=13) -> (element=w340:dbl)
          n185 = Index Array(array=w325, index=11) -> (element=w342:dbl)
          n186 = Index Array(array=w325, index=12) -> (element=w341:dbl)
          n187 = Compound Arithmetic op=ADD(w342, w341, w340) -> (w336:dbl)
          n188 = Multiply(x=w336, y=60.0) -> (x*y=w331:dbl)
          n189 = Index Array(array=w325, index=11) -> (element=w343:dbl)
          n190 = Multiply(x=w343, y=60.0) -> (x*y=w332:dbl)
          n191 = while {
            shift-right: [w573] -> _
            shift-left: w367 -> [w573]
            tunnel: w366 -> [w576]
            tunnel: [w576] -> w353
            tunnel: w332 -> [w572]
            tunnel: w343 -> [w575]
            i -> [w570]
            stop <- w568 stop-if-true
            # "Progress bar"
            n192 = call "ProgressBar.vi"("Time_end"=w572, "TimeBegin"=w573) -> ("TrueFalse"=w568:bool, "Stabilisation Bar"=w574:u8)
            n193 = Equal?(x=w570, y=0) -> (x = y?=w569:bool)
            n194 = case shown="True" w569 {
              frame False {
              }
              frame True {
                n195 = property on="OverviewTextFile" class="Path"() -> ("Value"=w579:path)  [unwired: 2 in, 2 out]
                n196 = call "UpdateTextFile_timestamp_string.vi"("string"="Waiting Dead Volume before data collection", "file path"=w579) -> ()  [unwired: 1 in]
              }
            }
            n197 = call "LightOn.vi"("Turns off when..."=w568) -> ("Light Indicator"=→"NMR Dead Volume":bool)
            n198 = property on="NMR Timesweep bar" class="Slide (strict)"("Value"=w574) -> ()  [unwired: 2 in, 2 out]
            n199 = local write "NMR Status"("Waiting Dead Volume... " ("NMR Status")) -> ()
            n200 = Wait (ms)(milliseconds to wait=u32 500) -> ()  [unwired: 1 out]
            "Waiting NMR" <- w575
          }
          n201 = local read "GPC use"() -> (w327:bool)
          n202 = case shown="True" w327 {
            tunnel: w367 -> [_ w394]
            tunnel: w366 -> [_ w393]
            tunnel: w347 -> [_ w384]
            tunnel: [_ w383] -> w346
            tunnel: w331 -> [_ w382]
            tunnel: [_ w379] -> w317
            tunnel: [_ w379] -> w316
            frame False {
              n203 = property on="Waiting GPC" class="DigNum (strict)"("Value"=0.0 ("Waiting GPC")) -> ()  [unwired: 2 in, 2 out]
              n204 = property on="GPC Timesweep" class="Slide (strict)"("Value"=u8 100 ("GPC Timesweep")) -> ()  [unwired: 2 in, 2 out]
              n205 = property on="Next injection" class="Slide (strict)"("Value"=u8 100 ("Next injection")) -> ()  [unwired: 2 in, 2 out]
              n206 = property on="GPC Samples" class="DigNum (strict)"("Value"=0.0 ("GPC Samples")) -> ()  [unwired: 2 in, 2 out]
              n207 = property on="GPC Status" class="Str"("Value"="No GPC measurement") -> ()  [unwired: 2 in, 2 out]
            }
            frame True {
              # "1) Calculate amount of samples\n2) N loop with N = amount of samples\n3) inject first sample and waits for interval (min)\n4) for N  = GPC samples: injections but case is False\n--> no waiting time"
              # "insert amount of GPC samples to the output array\ndo display in the interface"
              # "GPC Timesweep"
              n208 = while {
                shift-right: [w472] -> _
                shift-left: w394 -> [w472]
                tunnel: w382 -> [w471]
                tunnel: w393 -> [w474]
                tunnel: [w474] -> w392
                tunnel: [w468] -> w387
                stop <- w468 stop-if-true
                # "Progress bar"
                n209 = Divide(x=w471, y=60.0) -> (x/y=→"Waiting GPC":dbl)
                n210 = call "ProgressBar.vi"("Time_end"=w471, "TimeBegin"=w472) -> ("TrueFalse"=w468:bool, "Stabilisation Bar"=w466:u8)
                n211 = Wait (ms)(milliseconds to wait=u32 500) -> ()  [unwired: 1 out]
                n212 = call "LightOn.vi"("Turns off when..."=w468) -> ("Light Indicator"=→"GPC Dead Volume":bool)
                n213 = local write "GPC Timesweep"(w466) -> ()
                n214 = property on="GPC Status" class="Str"("Value"="Waiting for Dead Volume ... " ("GPC Status")) -> ()  [unwired: 2 in, 2 out]
              }
              n215 = flat-sequence {
                tunnel: w392 -> [w447]
                tunnel: [w447] -> w391
                tunnel: [w448] -> w390
                frame #0 {
                  n216 = Tick Count (ms)() -> (millisecond timer value=w448:u32)
                }
              }
              n217 = case shown="True" w387 {
                tunnel: [FALSE TRUE] -> w385
                tunnel: w392 -> [w462 w464]
                tunnel: [w462 w464] -> w386
                frame False {
                }
                frame True {
                }
              }
              n218 = local read "To... (min)"() -> (w381:dbl)
              n219 = Multiply(x=w381, y=60.0) -> (x*y=w389:dbl)
              n220 = while {
                shift-right: [w456] -> _
                shift-left: w390 -> [w456]
                tunnel: w389 -> [w455]
                tunnel: w391 -> [w458]
                tunnel: [w458] -> _
                tunnel: w381 -> [w449]
                i -> [w451]
                stop <- w453 stop-if-true
                # "Progress bar"
                n221 = local write "Waiting GPC"(w449) -> ()
                n222 = call "ProgressBar.vi"("Time_end"=w455, "TimeBegin"=w456) -> ("TrueFalse"=w453:bool, "Stabilisation Bar"=w454:u8)
                n223 = property on="GPC Timesweep" class="Slide (strict)"("Value"=w454) -> ()  [unwired: 2 in, 2 out]
                n224 = Equal?(x=0, y=w451) -> (x = y?=w452:bool)
                n225 = case shown="True" w452 {
                  frame False {
                  }
                  frame True {
                    n226 = property on="OverviewTextFile" class="Path"() -> ("Value"=w460:path)  [unwired: 2 in, 2 out]
                    n227 = call "UpdateTextFile_timestamp_string.vi"("string"="GPC timesweep started", "file path"=w460) -> ()  [unwired: 1 in]
                  }
                }
                n228 = Wait (ms)(milliseconds to wait=u32 500) -> ()  [unwired: 1 out]
                n229 = property on="GPC Status" class="Str"("Value"="Timesweep" ("String")) -> ()  [unwired: 2 in, 2 out]
              }
              n230 = case shown="True" w385 {
                tunnel: w386 -> [w400 w414]
                tunnel: [w399 w413] -> w379
                tunnel: [_ w407] -> w383
                tunnel: w384 -> [_ w409]
                tunnel: w381 -> [_ w405]
                tunnel: [TRUE FALSE] -> w378
                frame False {
                  n231 = for {
                    N: 0 -> [_]
                    tunnel: [w402] -> _ mode=indexing
                    tunnel: w400 -> [w401]
                    tunnel: [w401] -> w399 mode=indexing
                    i -> [w402]
                  }
                }
                frame True {
                  # "N = amount of GPC samples"
                  n232 = local read "GPC interval"() -> (w404:dbl)
                  n233 = call "RealAmountOfGPCSamples.vi"("GPC Interval"=w404, "tres2"=w405) -> ("Real amount of samples"=w410:dbl)
                  n234 = To Unsigned Byte Integer(number=w410) -> (unsigned 8bit integer=w412:u8)
                  "GPC Samples" <- w412
                  n235 = for {
                    N: w412 -> [w417]
                    tunnel: w414 -> [w419]
                    tunnel: [w418] -> w413 mode=indexing
                    i -> [w416]
                    n236 = Increment(x=w416) -> (x+1=w420:i32)
                    n237 = Equal?(x=w417, y=w420) -> (x = y?=w421:bool)
                    n238 = case shown="True" w421 {
                      tunnel: w419 -> [w435 w446]
                      tunnel: [w435 w446] -> w418
                      tunnel: w416 -> [w431 _]
                      frame False {
                        # "wait ms for next injection"
                        n239 = local read "GPC interval"() -> (w429:dbl)
                        n240 = Number To Decimal String(number=w431) -> (decimal integer string=w430:string)  [unwired: 1 in]
                        n241 = Multiply(x=60.0, y=w429) -> (x*y=w433:dbl)
                        n242 = Concatenate Strings("Waiting for injection ", w430) -> (w428:string)
                        n243 = Multiply(x=w433, y=1000.0) -> (x*y=w436:dbl)
                        n244 = flat-sequence {
                          tunnel: [w443] -> w434
                          frame #0 {
                            n245 = Tick Count (ms)() -> (millisecond timer value=w443:u32)
                          }
                        }
                        n246 = Wait (ms)(milliseconds to wait=w436) -> ()  [unwired: 1 out]
                        n247 = local write "Status injections"(w428) -> ()
                        n248 = while {
                          shift-right: [w440] -> _
                          shift-left: w434 -> [w440]
                          tunnel: w433 -> [w439]
                          stop <- w441 stop-if-true
                          n249 = call "ProgressBar.vi"("Time_end"=w439, "TimeBegin"=w440) -> ("TrueFalse"=w441:bool, "Stabilisation Bar"=w442:u8)
                          n250 = property on="Next injection" class="Slide (strict)"("Value"=w442) -> ()  [unwired: 2 in, 2 out]
                        }
                      }
                      frame True {
                        n251 = property on="GPC Status" class="Str"("Value"="Timesweep Done - Wait 3 seconds" ("String")) -> ()  [unwired: 2 in, 2 out]
                        n252 = Wait (ms)(milliseconds to wait=u32 3000) -> ()  [unwired: 1 out]
                      }
                    }
                    n253 = case shown="False" "GPC Injections" {
                      frame False {
                        n254 = property on="OverviewTextFile" class="Path"() -> ("Value"=w422:path)  [unwired: 2 in, 2 out]
                        n255 = call "UpdateTextFile_timestamp_string.vi"("string"="'GPC injections' off: no injection", "file path"=w422) -> ()  [unwired: 1 in]
                      }
                      frame True {
                        n256 = call "Inject VI.vi"("VISA Rescource name"="GPC connection port 2", "Delay before going back to load position (ms)"=u32 500 ("GPC: Delay before going\nback to load position (ms)")) -> ()
                        n257 = local read "OverviewTextFile"() -> (w424:path)
                        n258 = call "UpdateTextFile_timestamp_string.vi"("string"="GPC injection", "file path"=w424) -> ()  [unwired: 1 in]
                      }
                    }
                  }
                  n259 = property on="output array" class="Arr (strict)"() -> ("Value"=w406:dbl[])  [unwired: 2 in, 2 out]
                  n260 = Insert Into Array(array=w406, index=2, new element=w410) -> (w408:dbl[])
                  n261 = Build Array (concatenate)(w409, w408) -> (w407:dbl[][])
                }
              }
              n262 = call "LightOn.vi"("Turns off when..."=w378) -> ("Light Indicator"=→"GPC timesweep":bool)
              n263 = flat-sequence {
                tunnel: w379 -> [w396]
                tunnel: [w396] -> _
                frame #0 {
                  n264 = property on="GPC Status" class="Str"("Value"="Done" ("NMR Status")) -> ()  [unwired: 2 in, 2 out]
                }
              }
              n265 = property on="Status" class="Str"("Value"="Timesweep" ("Status")) -> ()  [unwired: 2 in, 2 out]
            }
          }
          "Reaction" <- w346
          n266 = property on="To... (min)" class="DigNum (strict)"() -> ("Value"=w324:dbl)  [unwired: 2 in, 2 out]
          n267 = flat-sequence {
            tunnel: [w500] -> w352
            tunnel: w353 -> [w500]
            tunnel: [w499] -> w351
            frame #0 {
              n268 = Tick Count (ms)() -> (millisecond timer value=w499:u32)
            }
          }
          n269 = Multiply(x=w324, y=60.0) -> (x*y=w350:dbl)
          n270 = while {
            shift-right: [w513] -> _
            shift-left: w351 -> [w513]
            tunnel: w352 -> [w518]
            tunnel: [w518] -> w348
            tunnel: w350 -> [w514]
            tunnel: w324 -> [w511]
            i -> [w507]
            stop <- w504 stop-if-true
            # "Start is scannumber when is 1. stop is calculting with NMR interval and \nto... (min)"
            # "Progress bar"
            n271 = call "ProgressBar.vi"("Time_end"=w514, "TimeBegin"=w513) -> ("TrueFalse"=w504:bool, "Stabilisation Bar"=w512:u8)
            n272 = Equal?(x=w507, y=0) -> (x = y?=w505:bool)
            n273 = property on="Waiting NMR" class="DigNum (strict)"("Value"=w511) -> ()  [unwired: 2 in, 2 out]
            n274 = property on="scan" class="DigNum (strict)"() -> ("Value"=w510:i32)  [unwired: 2 in, 2 out]
            n275 = property on="NMR Timesweep bar" class="Slide (strict)"("Value"=w512) -> ()  [unwired: 2 in, 2 out]
            n276 = property on="NMR interval" class="DigNum (strict)"() -> ("Value"=w502:dbl)  [unwired: 2 in, 2 out]
            n277 = call "Start_stopScan.vi"("NMR interval(sec)"=w502, "Count"=w507, "Scan#"=w510, "To...(min)"=w511) -> ("Stop Scan"=w508:dbl, "StartScan"=w509:dbl)
            "Stop Scan" <- w508
            "Start Scan" <- w509
            n278 = call "LightOn.vi"("Turns off when..."=w504) -> ("Light Indicator"=→"NMR timesweep":bool)
            n279 = Wait (ms)(milliseconds to wait=u32 500) -> ()  [unwired: 1 out]
            n280 = Build Array(w509) -> (w517:dbl[])
            n281 = case shown="True" w505 {
              frame False {
              }
              frame True {
                n282 = property on="OverviewTextFile" class="Path"() -> ("Value"=w521:path)  [unwired: 2 in, 2 out]
                n283 = call "UpdateTextFile_timestamp_string.vi"("string"="NMR timesweep Started", "file path"=w521) -> ()  [unwired: 1 in]
              }
            }
            n284 = Insert Into Array(array=w517, index=1, new element=w508) -> (→"output array":dbl[])
            n285 = local write "NMR Status"("Timesweep" ("NMR Status")) -> ()
          }
          n286 = flat-sequence {
            tunnel: w348 -> [w498]
            tunnel: [w498] -> _
            frame #0 {
              n287 = property on="OverviewTextFile" class="Path"() -> ("Value"=w496:path)  [unwired: 2 in, 2 out]
              n288 = property on="NMR Status" class="Str"("Value"="Done" ("NMR Status")) -> ()  [unwired: 2 in, 2 out]
              n289 = call "UpdateTextFile_timestamp_string.vi"("string"="NMR timesweep finished.", "file path"=w496) -> ()  [unwired: 1 in]
            }
          }
          n290 = call "Update_TimesweepDone_listbox.vi"("new array"=w346) -> ("New listbox"=w345:string[])  [unwired: 1 in]
          n291 = flat-sequence {
            tunnel: [w371] -> _
            tunnel: w316 -> [w371]
            tunnel: [TRUE] -> _
            frame #0 {
            }
          }
          n292 = property on="Finished_timesweeps" class="LstBox (strict)"("Item Names"=w345) -> ()  [unwired: 2 in, 2 out]
          n293 = property on="stop" class="Bool (strict)"() -> ("Value"=w330:bool)  [unwired: 2 in, 2 out]
        }
        n294 = flat-sequence {
          tunnel: w300 -> [w312]
          tunnel: [w312] -> _
          frame #0 {
            n295 = property on="Pump" class="VISAName"() -> ("Value"=w310:refnum<visa-resource-name>)  [unwired: 2 in, 2 out]
            n296 = call <instrlib>:"Initialize_Comm.vi"("Baud rate"=comm_rate_enum."9600", "Serial Port in"=w310) -> ("error out"=w308:errorcluster, "Serial Port out"=w307:refnum<visa-resource-name>)  [unwired: 8 in]
            n297 = call <instrlib>:"Stop.vi"("error in (no error)"=w308, "Serial Port in"=w307) -> ("error out"=w309:errorcluster)  [unwired: 8 in, 1 out]
            n298 = property on="Status" class="Str"("Value"="Stopped" ("Status")) -> ()  [unwired: 2 in, 2 out]
            n299 = flat-sequence {
              tunnel: w309 -> [w314]
              tunnel: [w314] -> _
              frame #0 {
                n300 = Wait (ms)(milliseconds to wait=u32 1000) -> ()  [unwired: 1 out]
              }
            }
          }
        }
        n301 = while {
          stop <- w301 stop-if-true
          n302 = case shown="True" "Insert Comment" {
            tunnel: "Cooment" -> [_ w305]
            frame False {
            }
            frame True {
              n303 = local read "Comments file"() -> (w304:path)
              n304 = call "UpdateTextFile_timestamp_string.vi"("string"=w305, "file path"=w304) -> ()  [unwired: 1 in]
              n305 = invoke on="Cooment" class="Str" method="Reinit To Default"() -> ()  [unwired: 3 in, 3 out]
              "Last Comment" <- w305
            }
          }
          n306 = property on="stop" class="Bool (strict)"() -> ("Value"=w301:bool)  [unwired: 2 in, 2 out]
        }
      }
    }
    n307 = property on="stop" class="Bool (strict)"() -> ("Value"=w264:bool)  [unwired: 2 in, 2 out]
  }
  n308 = property on="Finished_timesweeps" class="LstBox (strict)"("Item Names"=string[] [""]) -> ()  [unwired: 2 in, 2 out]
  "Reactor Volume" <- 0.0 ("Reactor Volume")
